vi "生成-报警记录缓存数据文件-分类计时版.vi"(8 "缓存绘图数据":cluster{"X":timestamp[], "Y":dbl[]}, 9 "限值":T1, 10 "探头信息":string, 11 "探头地址":i32) -> ()   [LabVIEW 2017]
panel:
  out "开始时间2":string
  out "开始时间1":string
  out "开始2":timestamp
  out "开始1":timestamp
  out "最大值":string
  out "限值2":string
  out "限值1":string
  out "实时曲线":cluster{"X":timestamp[], "Y":dbl[]}[](graph)
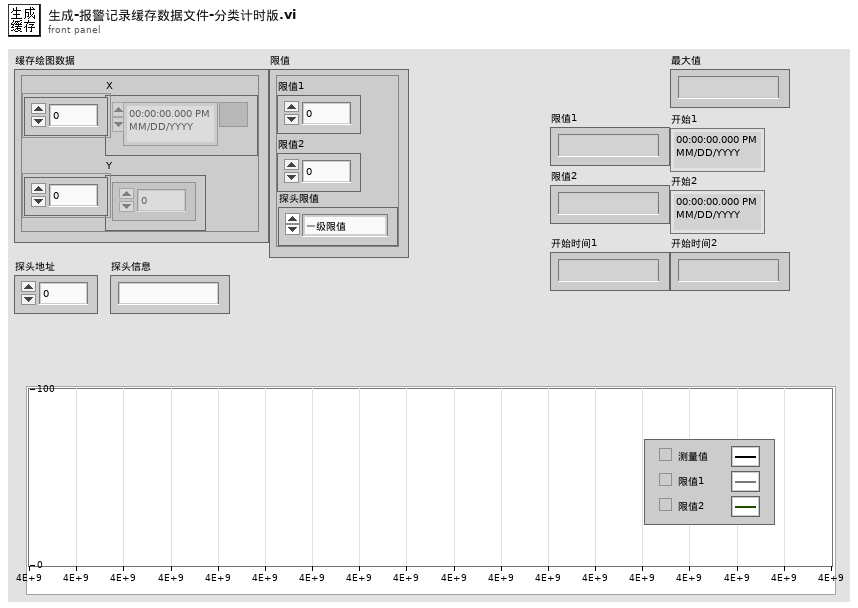
[diagram p1: front panel]
types:
  T1 = cluster{"限值1":dbl, "限值2":dbl, "探头限值":enum16{"一级限值", "二级限值"}}
  T2 = cluster{"限值":string, "报警时长":string, "最大值":string, "开始时间":string}
  T3 = cluster{"限值":string, "报警时长":string, "最大值":string, "开始时间":string}[]
  T4 = cluster{"实时曲线":cluster{"X":timestamp[], "Y":dbl[]}[], "书签-键-值":string[][]}
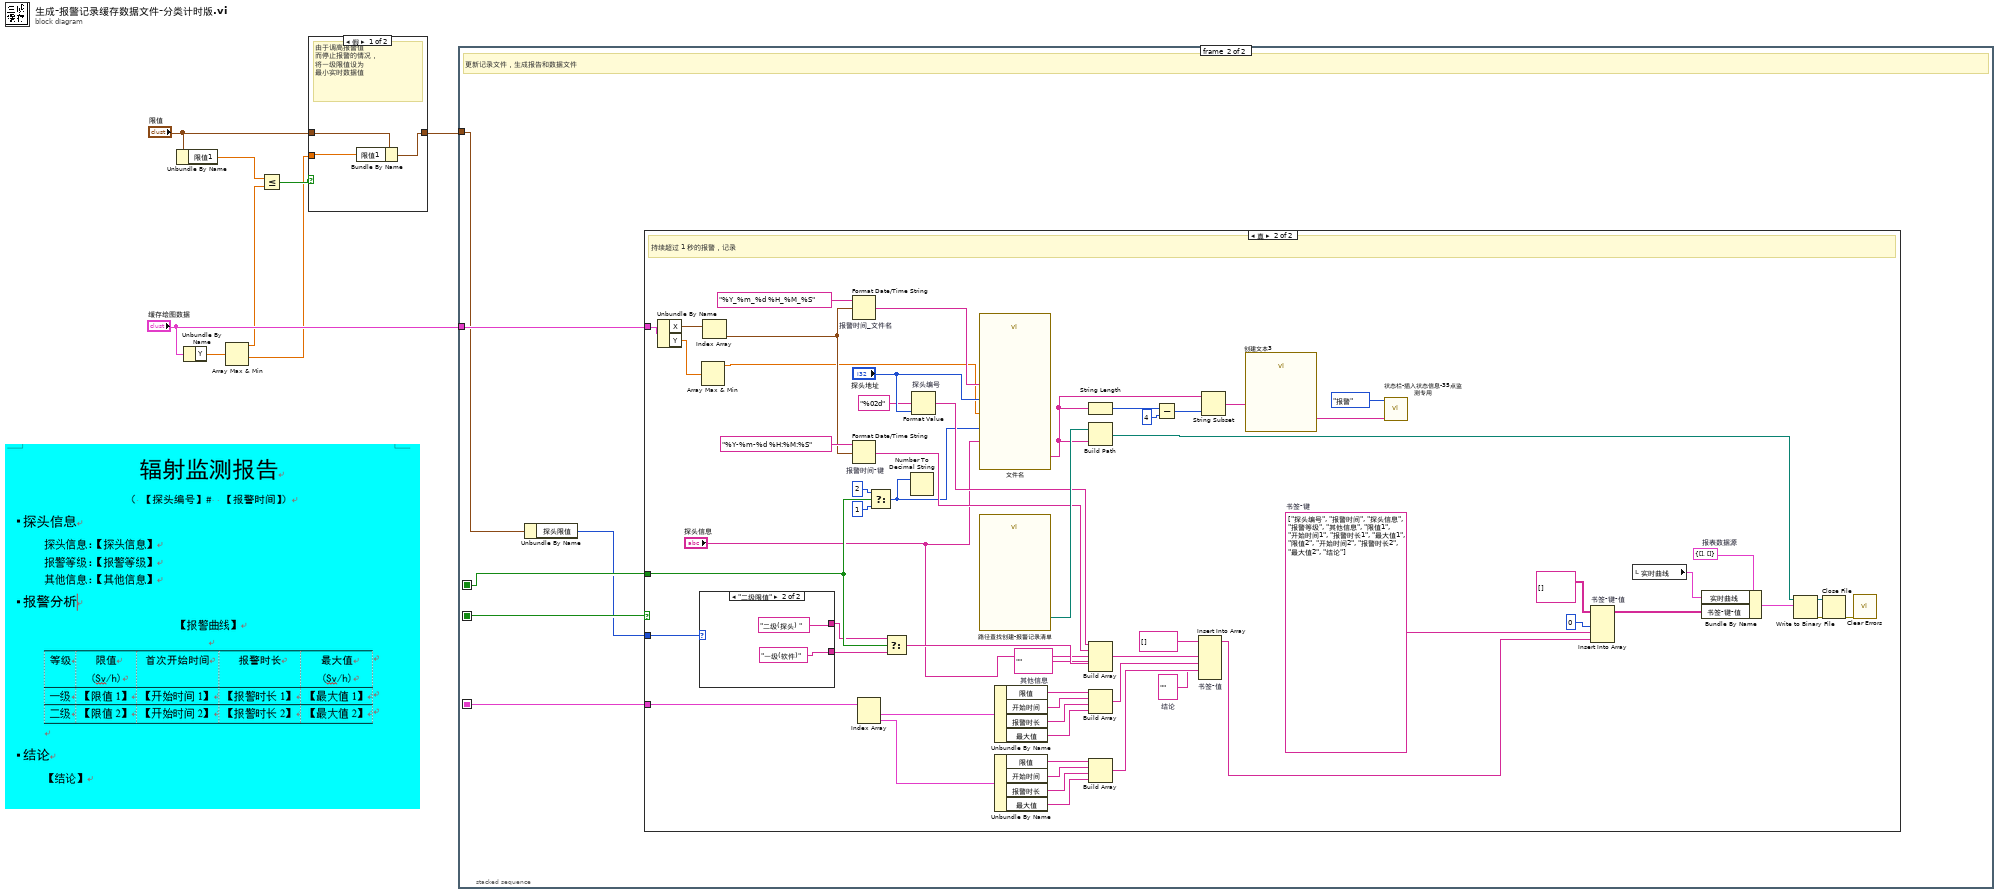
[diagram p0: block diagram]
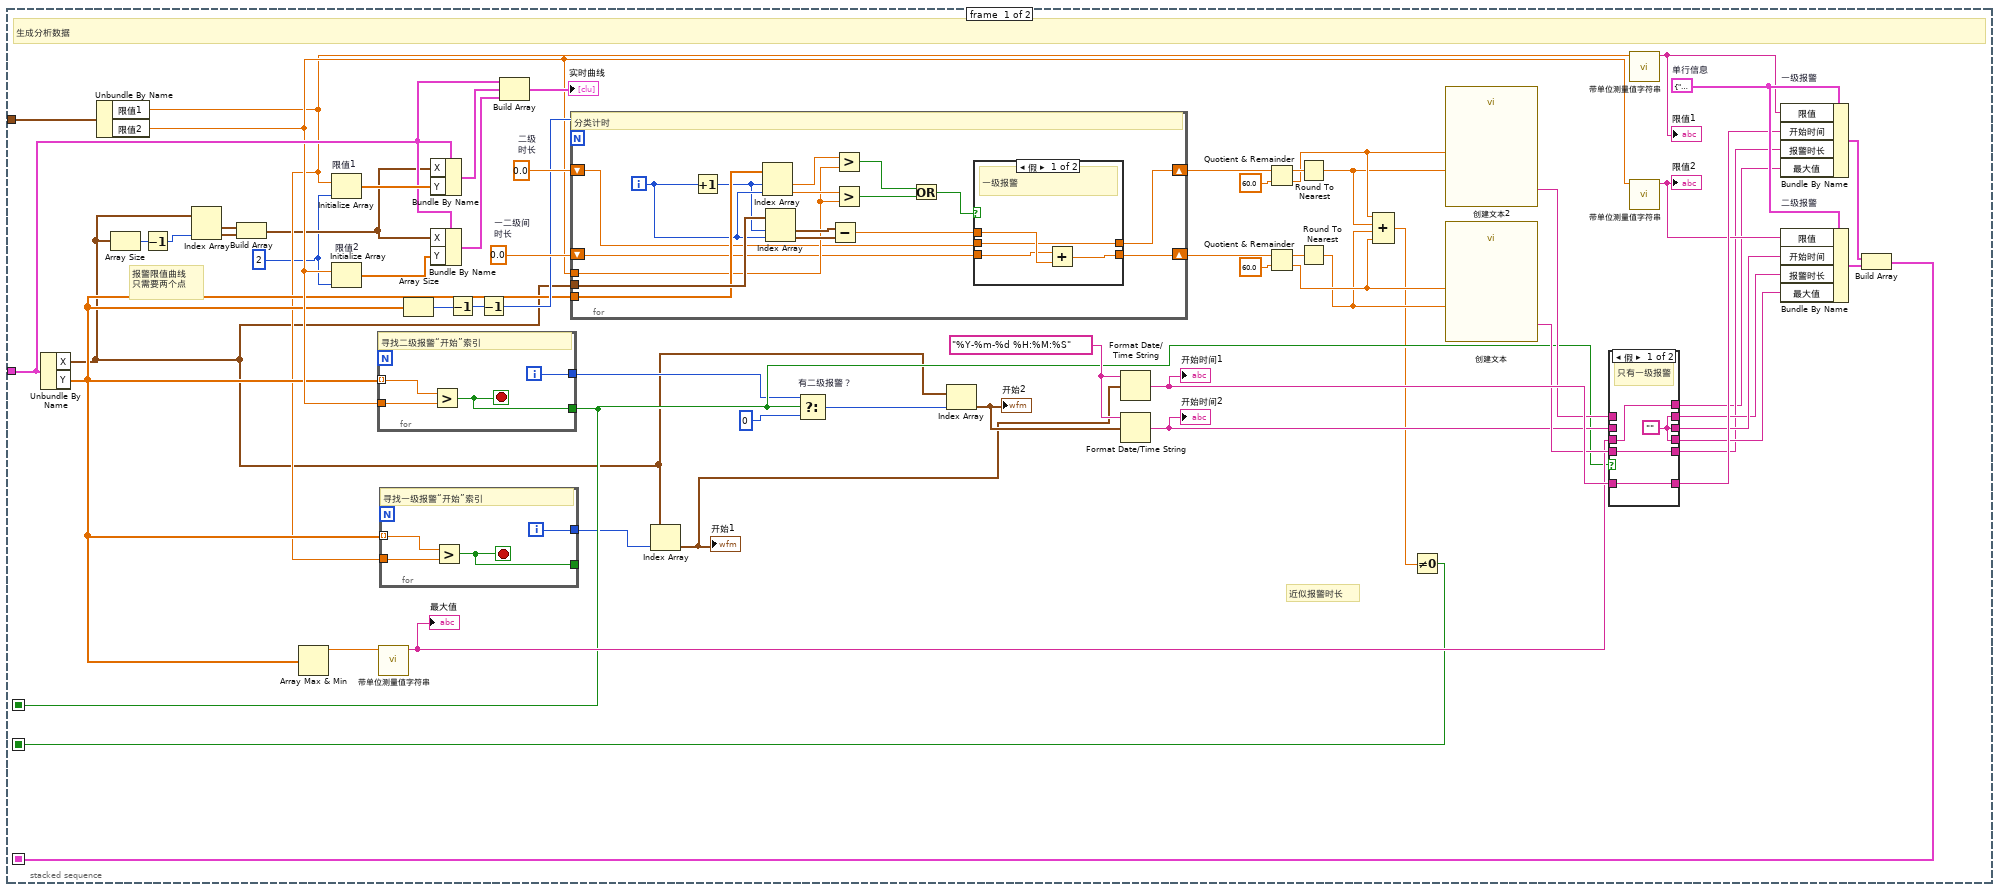
[diagram p3: hidden frame]
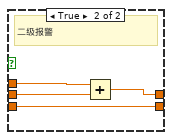
[diagram p4: hidden frame]
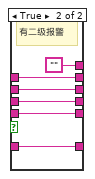
[diagram p5: hidden frame]
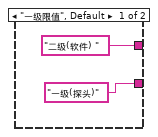
[diagram p7: hidden frame]
diagram:
  n1 = Unbundle By Name("限值") -> ("限值1"=w6:dbl)
  n2 = Unbundle By Name("缓存绘图数据") -> ("Y"=w7:dbl[])
  n3 = Array Max & Min(array=w7) -> (max value=w5:dbl, min value=w1:dbl)  [unwired: 2 out]
  n4 = Less Or Equal?(x=w6, y=w5) -> (x <= y?=w4:bool)
  n5 = case shown="假" w4 {
    tunnel: [w9 w12] -> w3
    tunnel: "限值" -> [w11 w12]
    tunnel: w1 -> [w10 _]
    frame False {
      # "由于调高报警值\n而停止报警的情况，\n将一级限值设为\n最小实时数据值"
      n6 = Bundle By Name(cluster=w11, "限值1"=w10) -> (w9:T1)
    }
    frame True {
    }
  }
  n7 = stacked-sequence {
    seq-local: [w47 _] -> [_ w119]
    seq-local: [w45 _] -> [_ w120]
    seq-local: [w20 _] -> [_ w118]
    tunnel: "缓存绘图数据" -> [w46 w121]
    tunnel: w3 -> [w30 w117]
    frame #0 {
      w13 = 2 ("维数大小")
      w40 = 0.0  # 二级 时长
      w41 = 0.0  # 一二级间 时长
      w63 = T2 {"限值"="", "报警时长"="", "最大值"="", "开始时间"=""}  # 单行信息
      w60 = "%Y-%m-%d %H:%M:%S" ("时间格式字符串(%c)")
      # "报警限值曲线\n只需要两个点"
      # "近似报警时长"
      # "生成分析数据"
      n8 = Unbundle By Name(w46) -> ("X"=w15:timestamp[], "Y"=w29:dbl[])
      n9 = Unbundle By Name(w30) -> ("限值1"=w28:dbl, "限值2"=w37:dbl)
      n10 = Array Size(array=w15) -> (size(s)=w19:i32)
      n11 = Decrement(x=w19) -> (x-1=w18:i32)
      n12 = Index Array(array=w15, index #2=w18) -> (element #1=w17:timestamp, element #2=w16:timestamp)  [unwired: 1 in]
      n13 = Build Array(w17, w16) -> (w14:timestamp[])
      n14 = Array Max & Min(array=w29) -> (max value=w66:dbl)  [unwired: 3 out]
      n15 = Initialize Array "限值1"(w28, w13) -> (w71:dbl[])
      n16 = Initialize Array "限值2"(w37, w13) -> (w70:dbl[])
      n17 = for {
        tunnel: w29 -> [w115] mode=indexing
        tunnel: w37 -> [w114]
        tunnel: [w113] -> w44
        tunnel: [w112] -> w45
        i -> [w113]
        stop <- w112 stop-if-true
        # "寻找二级报警“开始”索引"
        n18 = Greater?(x=w115, y=w114) -> (0:w112:bool)
      }
      n19 = call "带单位测量值字符串.vi"("测量值"=w66) -> ("结果"=w55:string)  [unwired: 10 in]
      "最大值" <- w55
      n20 = for {
        tunnel: w29 -> [w76] mode=indexing
        tunnel: w28 -> [w75]
        tunnel: [w74] -> w27
        tunnel: [w73] -> _
        i -> [w74]
        stop <- w73 stop-if-true
        # "寻找一级报警“开始”索引"
        n21 = Greater?(x=w76, y=w75) -> (0:w73:bool)
      }
      n22 = Array Size(array=w29) -> (size(s)=w72:i32)
      n23 = Bundle By Name(cluster=w46, "X"=w14, "Y"=w71) -> (w69:cluster{"X":timestamp[], "Y":dbl[]})
      n24 = Bundle By Name(cluster=w46, "X"=w14, "Y"=w70) -> (w68:cluster{"X":timestamp[], "Y":dbl[]})
      n25 = Decrement(x=w72) -> (x-1=w39:i32)
      n26 = Decrement(x=w39) -> (x-1=w38:i32)
      n27 = Build Array(w46, w69, w68) -> (→"实时曲线":cluster{"X":timestamp[], "Y":dbl[]}[])
      n28 = for {
        N: w38 -> [_]
        shift-right: [w80] -> w35
        shift-left: w40 -> [w82]
        shift-right: [w79] -> w36
        shift-left: w41 -> [w78]
        tunnel: w15 -> [w93]
        tunnel: w29 -> [w90]
        tunnel: w37 -> [w86]
        i -> [w89]
        # "分类计时"
        n29 = Increment(x=w89) -> (x+1=w77:i32)
        n30 = Index Array(array=w90, index #1=w77, index #2=w89) -> (element #1=w88:dbl, element #2=w87:dbl)
        n31 = Index Array(array=w93, index #1=w77, index #2=w89) -> (element #1=w92:timestamp, element #2=w91:timestamp)
        n32 = Subtract(x=w92, y=w91) -> (x-y=w81:dbl)
        n33 = Greater?(x=w88, y=w86) -> (0:w84:bool)
        n34 = Greater?(x=w87, y=w86) -> (0:w85:bool)
        n35 = Or(x=w84, y=w85) -> (x .or. y?=w83:bool)
        n36 = case shown="假" w83 {
          tunnel: w82 -> [w94 w100]
          tunnel: w81 -> [w97 w101]
          tunnel: [w94 w99] -> w80
          tunnel: [w95 w98] -> w79
          tunnel: w78 -> [w96 w98]
          frame False {
            # "一级报警"
            n37 = Add(x=w96, y=w97) -> (x+y=w95:dbl)
          }
          frame True {
            # "二级报警"
            n38 = Add(x=w101, y=w100) -> (x+y=w99:dbl)
          }
        }
      }
      n39 = Index Array(array=w15, index=w27) -> (element=w26:timestamp)
      "开始1" <- w26
      n40 = Select "有二级报警？"(t=w44, s=w45, f=0) -> (s? t:f=w42:i32)
      n41 = Index Array(array=w15, index=w42) -> (element=w59:timestamp)
      "开始2" <- w59
      n42 = Format Date/Time String(time format string (%c)=w60, seconds (now)=w26) -> (date/time string=w57:string)  [unwired: 1 in]
      "开始时间1" <- w57
      n43 = Format Date/Time String(time format string (%c)=w60, seconds (now)=w59) -> (date/time string=w49:string)  [unwired: 1 in]
      "开始时间2" <- w49
      n44 = Quotient & Remainder(x=w35, y=60.0) -> (x-y*floor(x/y)=w62:dbl, floor(x/y)=w25:dbl)
      n45 = Quotient & Remainder(x=w36, y=60.0) -> (x-y*floor(x/y)=w64:dbl, floor(x/y)=w23:dbl)
      n46 = Round To Nearest(number=w62) -> (nearest integer value=w24:dbl)
      n47 = Round To Nearest(number=w64) -> (nearest integer value=w22:dbl)
      n48 = Compound Arithmetic op=ADD(w25, w24, w22, w23) -> (w21:dbl)
      n49 = Not Equal To 0?(x=w21) -> (x != 0?=w20:bool)
      n50 = call "创建文本2"("分"=w25, "秒"=w24) -> ("Result"=w48:string)  [unwired: 12 in, 1 out]
      n51 = call "创建文本"("分"=w23, "秒"=w22) -> ("Result"=w56:string)  [unwired: 12 in, 1 out]
      n52 = case shown="假" w45 {
        tunnel: [w105 w110] -> w58
        tunnel: w57 -> [w105 w110]
        tunnel: [w104 w109] -> w32
        tunnel: w56 -> [w104 w109]
        tunnel: w55 -> [w103 w106]
        tunnel: [w103 ""] -> w31
        tunnel: [w102 w108] -> w50
        tunnel: [w102 w107] -> w34
        tunnel: [w102 w106] -> w33
        tunnel: w49 -> [_ w108]
        tunnel: w48 -> [_ w107]
        frame False {
          w102 = ""
          # "只有一级报警"
        }
        frame True {
          # "有二级报警"
        }
      }
      n53 = call "带单位测量值字符串.vi"("测量值"=w28) -> ("结果"=w54:string)  [unwired: 10 in]
      "限值1" <- w54
      n54 = call "带单位测量值字符串.vi"("测量值"=w37) -> ("结果"=w53:string)  [unwired: 10 in]
      "限值2" <- w53
      n55 = Bundle By Name "一级报警"(cluster=w63, "限值"=w54, "开始时间"=w58, "报警时长"=w32, "最大值"=w31) -> (w52:T2)
      n56 = Bundle By Name "二级报警"(cluster=w63, "限值"=w53, "开始时间"=w50, "报警时长"=w34, "最大值"=w33) -> (w51:T2)
      n57 = Build Array(w52, w51) -> (w47:T3)
    }
    frame #1 {
      # "更新记录文件，生成报告和数据文件"
      n58 = Unbundle By Name(w117) -> ("探头限值"=w116:enum16{"一级限值", "二级限值"})
      n59 = case "条件结构" shown="真" w118 {
        tunnel: w121 -> [_ w179]
        tunnel: w120 -> [_ w171]
        tunnel: w119 -> [_ w168]
        tunnel: w116 -> [_ w124]
        frame False {
          # "持续不到 1 秒，不记录"
        }
        frame True {
          w150 = T4 {"实时曲线"=[], "书签-键-值"=[]}  # 报表数据源
          w152 = string[] ["探头编号", "报警时间", "探头信息", "报警等级", "其他信息", "限值1", "开始时间1", "报警时长1", "最大值1", "限值2", "开始时间2", "报警时长2", "最大值2", "结论"]  # 书签-键
          w155 = ""  # 结论
          w169 = ""  # 其他信息
          # "持续超过 1 秒的报警，记录"
          n60 = Unbundle By Name(w179) -> ("X"=w178:timestamp[], "Y"=w133:dbl[])
          n61 = case shown="\"二级限值\"" w124 {
            tunnel: ["二级(软件) " ("格式字符串") "二级(探头) " ("格式字符串")] -> w122
            tunnel: ["一级(探头)" ("格式字符串") "一级(软件)" ("格式字符串")] -> w123
            frame "一级限值", Default {
            }
            frame "二级限值" {
            }
          }
          n62 = Array Max & Min(array=w133) -> (max value=w132:dbl)  [unwired: 3 out]
          n63 = Index Array(array=w178) -> (element=w144:timestamp)  [unwired: 1 in]
          n64 = Format Date/Time String "报警时间_文件名"(time format string (%c)="%Y_%m_%d %H_%M_%S" ("时间格式字符串(%c)"), seconds (now)=w144) -> (date/time string=w143:string)  [unwired: 1 in]
          n65 = Format Date/Time String "报警时间-键"(time format string (%c)="%Y-%m-%d %H:%M:%S" ("时间格式字符串(%c)"), seconds (now)=w144) -> (date/time string=w147:string)  [unwired: 1 in]
          n66 = Index Array(array=w168) -> (element #1=w167:T2, element #2=w166:T2)  [unwired: 2 in]
          n67 = Select(t=2, s=w171, f=1) -> (s? t:f=w131:i32)
          n68 = Select(t=w122, s=w171, f=w123) -> (s? t:f=w170:string)
          n69 = Number To Decimal String(number=w131) -> ()  [unwired: 1 in, 1 out]
          n70 = Format Value "探头编号"(format string="%02d" ("格式字符串"), value (0)="探头地址") -> (output string=w146:string)  [unwired: 1 in]
          n71 = call "文件名"("最大值"=w132, "时间"=w143, "探头地址XX"="探头地址", "探头名称"="探头信息", "报警等级"=w131) -> ("Result"=w137:string)  [unwired: 9 in, 1 out]
          n72 = call "路径查找创建-报警记录清单.vi"() -> ("缓存数据文件夹"=w176:path)  [unwired: 8 in, 11 out]
          n73 = Unbundle By Name(w167) -> ("限值"=w165:string, "开始时间"=w164:string, "报警时长"=w135:string, "最大值"=w134:string)
          n74 = Unbundle By Name(w166) -> ("限值"=w163:string, "开始时间"=w162:string, "报警时长"=w161:string, "最大值"=w160:string)
          n75 = String Length(string=w137) -> (length=w140:i32)
          n76 = Build Path(base path=w176, name or relative path=w137) -> (appended path=w125:path)
          n77 = Build Array(w146, w147, "探头信息", w170, w169) -> (w159:string[])
          n78 = Build Array(w165, w164, w135, w134) -> (w157:string[])
          n79 = Build Array(w163, w162, w161, w160) -> (w156:string[])
          n80 = Subtract(x=w140, y=4) -> (x-y=w138:i32)
          n81 = Insert Into Array "书签-值"(array=string[] [] ("数组"), new element #1=w159, new element #2=w157, new element #3=w156, new element #4=w155) -> (w151:string[])  [unwired: 1 in]
          n82 = String Subset(string=w137, length (rest)=w138) -> (substring=w136:string)  [unwired: 1 in]
          n83 = call "创建文本3"("文件名"=w136) -> ("Result"=w141:string)  [unwired: 13 in, 1 out]
          n84 = call "状态栏-插入状态信息-35点监测专用.vi"("消息内容"=w141, "状态类型"=enum16{"全部", "报警", "通信", "设置"}."报警") -> ()  [unwired: 10 in]
          n85 = Insert Into Array "书签-键-值"(array=string[][] [] ("数组"), index (col)=0 ("禁用的索引 (列)"), new element #1=w152, new element #2=w151) -> (w148:string[][])  [unwired: 1 in]
          n86 = local read "实时曲线"() -> (w149:cluster{"X":timestamp[], "Y":dbl[]}[])
          n87 = Bundle By Name(cluster=w150, "实时曲线"=w149, "书签-键-值"=w148) -> (w126:T4)
          n88 = Write to Binary File(file (use dialog)=w125, data=w126) -> (refnum out=w128:refnum<file>, error out=w129:errorcluster)  [unwired: 4 in, 1 out]
          n89 = Close File(refnum=w128, error in=w129) -> (error out=w127:errorcluster)  [unwired: 1 out]
          n90 = call <vilib>:"Clear Errors.vi"("error in (no error)"=w127) -> ()  [unwired: 5 in, 2 out]
        }
      }
    }
  }
